vi "Detect Song.vi"(0 "Audio Array":dbl[](array[numeric])=array[4410 elements], 2 "Detect Parameters":T1={"High Freq. Song"=7000.0, "Low Freq. Song"=4000.0, "High Freq. Noise"=200.0, "Low Freq. Noise"=50.0, "Samples Per Channel"=4410.0, "SampClk.Rate"=44150.11037527594, "# Crossing per Samples\nSong Detected (ON)"=3.0, "# Crossing per Samples\nSong Completed (OFF)"=0.0, "Ratio Threshold"=3.0, "Dectect window"=6}, 6 "Dbl Shift In":dbl[](array[numeric])=array[44100 elements], 7 "Bool Shift In":bool[](array[boolean])=[FALSE, FALSE, FALSE, FALSE, FALSE, FALSE]) -> (12 "Dbl Shift Out":dbl[](array[numeric]), 13 "Bool Shift Out":bool[](array[boolean]), 14 "Buffered Audio To Save":dbl[](array[numeric]), 15 "Song Detect":bool, 18 "Current Ratio":dbl=0.016229870659951417)   [LabVIEW 2016]
uses:
  <vilib>/Analysis/baseanly.llb/Real Dot Product.vi
  <vilib>/Analysis/3filter.llb/Butterworth Filter (DBL).vi
  <vilib>/Analysis/NI_AALBase.lvlib
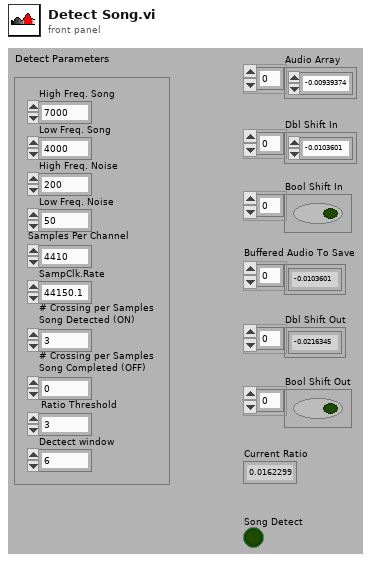
[diagram p1: front panel]
types:
  T1 = cluster{"High Freq. Song":dbl, "Low Freq. Song":dbl, "High Freq. Noise":dbl, "Low Freq. Noise":dbl, "Samples Per Channel":dbl, "SampClk.Rate":dbl, "# Crossing per Samples\nSong Detected (ON)":dbl, "# Crossing per Samples\nSong Completed (OFF)":dbl, "Ratio Threshold":dbl, "Dectect window":i32}
  T2 = enum32{"Lowpass", "Highpass", "Bandpass", "Bandstop"}
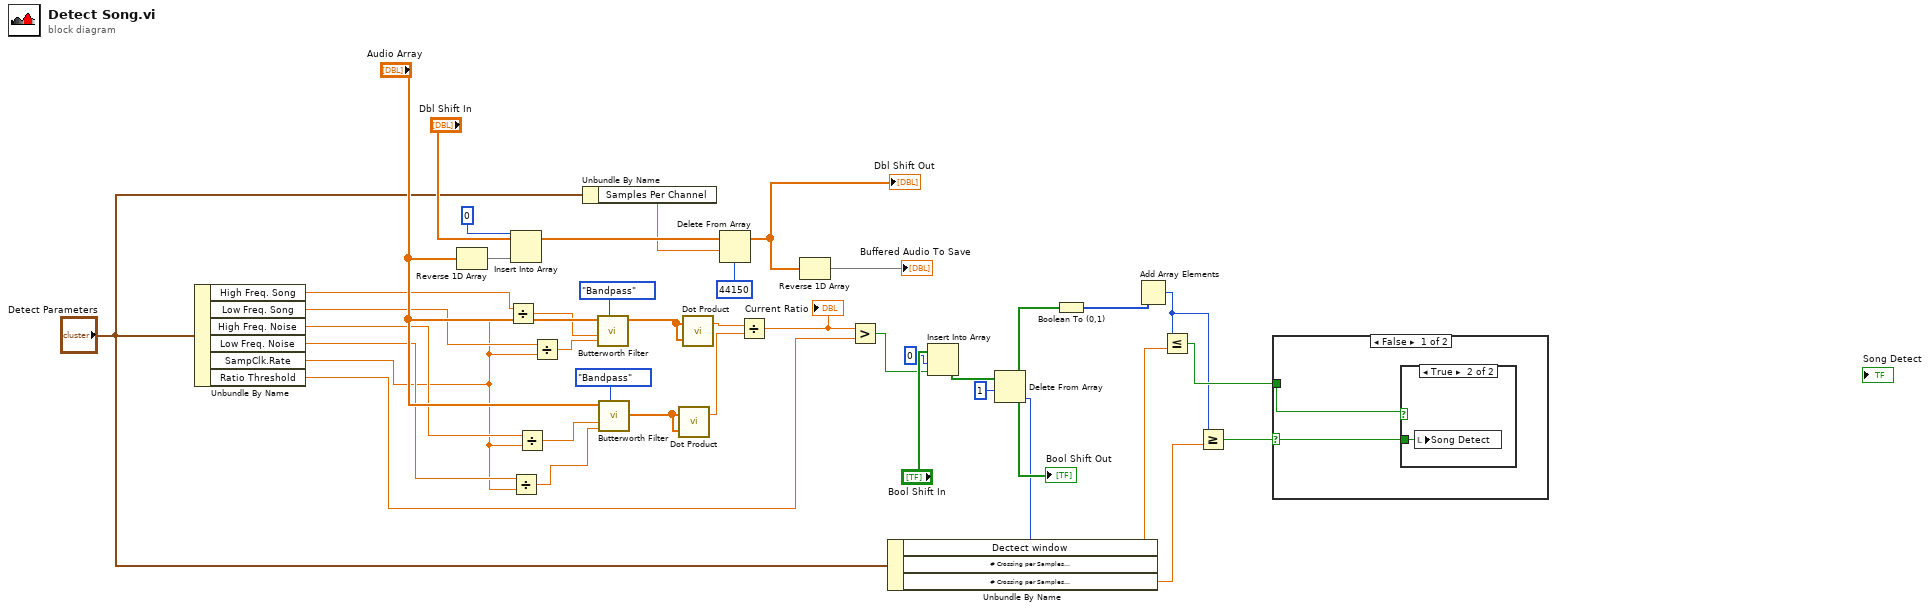
[diagram p0: block diagram]
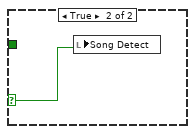
[diagram p3: hidden frame]
diagram:
  n1 = Unbundle By Name("Detect Parameters") -> ("High Freq. Song"=w11:dbl, "Low Freq. Song"=w10:dbl, "High Freq. Noise"=w9:dbl, "Low Freq. Noise"=w8:dbl, "SampClk.Rate"=w3:dbl, "Ratio Threshold"=w2:dbl)
  n2 = Reverse 1D Array(array="Audio Array") -> (reversed array=w25:dbl[])
  n3 = Divide(x=w11, y=w3) -> (x/y=w28:dbl)
  n4 = Insert Into Array(array="Dbl Shift In", index=0, new element=w25) -> (w24:dbl[])
  n5 = Divide(x=w8, y=w3) -> (x/y=w30:dbl)
  n6 = Divide(x=w9, y=w3) -> (x/y=w38:dbl)
  n7 = Divide(x=w10, y=w3) -> (x/y=w29:dbl)
  n8 = Unbundle By Name("Detect Parameters") -> ("Samples Per Channel"=w4:dbl)
  n9 = call-poly <vilib>:"Butterworth Filter.vi"("filter type"=T2."Bandpass", "low cutoff freq: fl"=w29, "high cutoff freq: fh"=w28, "X"="Audio Array") -> ("Filtered X"=w35:dbl[])  [unwired: 3 in, 2 out]
  n10 = call-poly <vilib>:"Butterworth Filter.vi"("filter type"=T2."Bandpass", "low cutoff freq: fl"=w30, "high cutoff freq: fh"=w38, "X"="Audio Array") -> ("Filtered X"=w34:dbl[])  [unwired: 3 in, 2 out]
  n11 = call-poly <vilib>:"Dot Product.vi"("Y Vector"=w34, "X Vector"=w34) -> ("X * Y"=w33:dbl)  [unwired: 1 out]
  n12 = call-poly <vilib>:"Dot Product.vi"("Y Vector"=w35, "X Vector"=w35) -> ("X * Y"=w32:dbl)  [unwired: 1 out]
  n13 = Delete From Array(array=w24, length=w4, index=44150) -> (array with subset deleted=w27:dbl[])  [unwired: 1 out]
  "Dbl Shift Out" <- w27
  n14 = Divide(x=w32, y=w33) -> (x/y=w31:dbl)
  "Current Ratio" <- w31
  n15 = Reverse 1D Array(array=w27) -> (reversed array=→"Buffered Audio To Save":dbl[])
  n16 = Greater?(x=w31, y=w2) -> (0:w15:bool)
  n17 = Unbundle By Name("Detect Parameters") -> ("Dectect window"=w1:i32, "# Crossing per Samples\nSong Completed (OFF)"=w7:dbl, "# Crossing per Samples\nSong Detected (ON)"=w6:dbl)
  n18 = Insert Into Array(array="Bool Shift In", index=0, new element=w15) -> (w16:bool[])
  n19 = Delete From Array(array=w16, length=1, index=w1) -> (array with subset deleted=w37:bool[])  [unwired: 1 out]
  "Bool Shift Out" <- w37
  n20 = Boolean To (0,1)(Boolean=w37) -> (0, 1=w18:i16[])
  n21 = Add Array Elements(numeric array=w18) -> (sum=w20:i16)
  n22 = Less Or Equal?(x=w20, y=w7) -> (x <= y?=w21:bool)
  n23 = Greater Or Equal?(x=w20, y=w6) -> (x >= y?=w19:bool)
  n24 = case shown="False" w19 {
    selector: w19 -> [w41 w44]
    tunnel: w21 -> [w42 _]
    frame False {
      n25 = case shown="True" w42 {
        tunnel: w41 -> [_ w43]
        frame False {
        }
        frame True {
          n26 = local write "Song Detect"(w43) -> ()
        }
      }
    }
    frame True {
      n27 = local write "Song Detect"(w44) -> ()
    }
  }
